vi "Controller_Heating_Test.vi"() -> ()   [LabVIEW 2010]
uses:
  labbCAN_Bus_API/labbCAN_Bus_API.lvlib
  labbCAN_Controller_API/labbCAN_Controller_API.lvlib
panel:
  out "Actual Value":dbl
  in  "Stopp":bool
  out "error out":errorcluster caption="Fehler (Ausgang)"
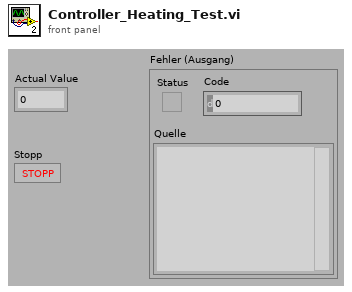
[diagram p1: front panel]
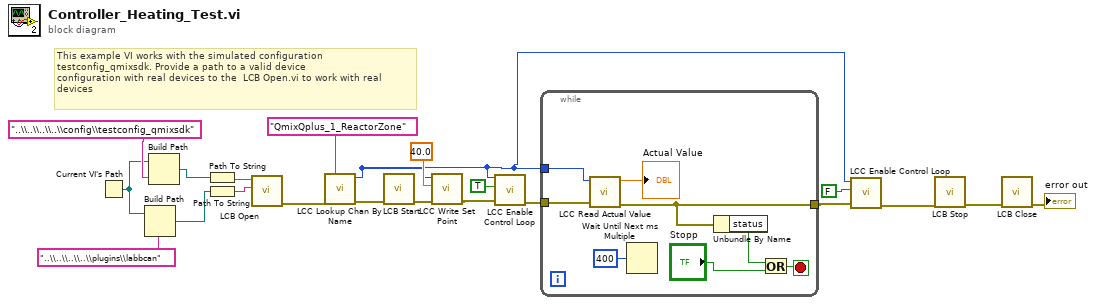
[diagram p0: block diagram]
diagram:
  # "This example VI works with the simulated configuration\ntestconfig_qmixsdk. Provide a path to a valid device\nconfiguration with real devices to the  LCB Open.vi to work with real\ndevices"
  n1 = Current VI's Path() -> (path=w10:path)
  n2 = Build Path(base path=w10, name or relative path="..\\..\\..\\..\\plugins\\labbcan" ("Name oder relativer Pfad")) -> (appended path=w18:path)
  n3 = Build Path(base path=w10, name or relative path="..\\..\\..\\..\\config\\testconfig_qmixsdk" ("Name oder relativer Pfad")) -> (appended path=w4:path)
  n4 = Path To String(path=w4) -> (string=w5:string)
  n5 = Path To String(path=w18) -> (string=w16:string)
  n6 = call "LCB Open.vi"("PluginSearchPath"=w16, "Device Configuration Path"=w5) -> ("error out"=w9:errorcluster)  [unwired: 9 in]
  n7 = call "LCC Lookup Chan By Name.vi"("error in (no error)"=w9, "Channel Name"="QmixQplus_1_ReactorZone") -> ("error out"=w14:errorcluster, "Channel Handle"=w6:i64)  [unwired: 8 in]
  n8 = call "LCB Start.vi"("error in (no error)"=w14) -> ("error out"=w13:errorcluster)  [unwired: 10 in]
  n9 = call "LCC Write Set Point.vi"("error in (no error)"=w13, "Setpoint"=40.0, "Channel Handle"=w6) -> ("error out"=w3:errorcluster)  [unwired: 8 in]
  n10 = call "LCC Enable Control Loop.vi"("error in (no error)"=w3, "Enable"=TRUE, "ChanHdl"=w6) -> ("error out"=w11:errorcluster)  [unwired: 8 in]
  n11 = while {
    tunnel: w11 -> [w28]
    tunnel: [w26] -> w2
    tunnel: w6 -> [w22]
    stop <- w23 stop-if-true
    n12 = call "LCC Read Actual Value.vi"("error in (no error)"=w28, "Channel Handle"=w22) -> ("error out"=w26:errorcluster, "Actual Value"=→"Actual Value":dbl)  [unwired: 8 in]
    n13 = Wait Until Next ms Multiple(millisecond multiple=u32 400 ("Vielfache von ms")) -> ()  [unwired: 1 out]
    n14 = Unbundle By Name(w26) -> ("status"=w25:bool)
    n15 = Or(x=w25, y="Stopp") -> (x .or. y?=w23:bool)
  }
  n16 = call "LCC Enable Control Loop.vi"("error in (no error)"=w2, "Enable"=FALSE, "ChanHdl"=w6) -> ("error out"=w7:errorcluster)  [unwired: 8 in]
  n17 = call "LCB Stop.vi"("error in (no error)"=w7) -> ("error out"=w20:errorcluster)  [unwired: 10 in]
  n18 = call "LCB Close.vi"("error in (no error)"=w20) -> ("error out"=→"error out":errorcluster)  [unwired: 10 in]
